vi "Crop Video Size Utility.vi"() -> ()   [LabVIEW 2017]
uses:
  LabVIEW/Controls/Frame Grabber Data.ctl
  <vilib>/userdefined/High Color/IMAQdx.ctl
  <vilib>/vision/Image Controls.llb/IMAQ Image.ctl
  <vilib>/vision/Avi.llb/IMAQ AVI2 Refnum.ctl
  LabVIEW/Controls/Rigid Body Info.ctl
  LabVIEW/Controls/Position.ctl
  LabVIEW/Controls/Orientation.ctl
  LabVIEW/Controls/Refnums.ctl
  LabVIEW/Controls/Recording Settings.ctl
  LabVIEW/Controls/Operator Settings.ctl
  LabVIEW/Controls/Operator.ctl
  LabVIEW/Controls/Dimensions.ctl
  LabVIEW/Controls/Room Dimensions.ctl
  <vilib>/vision/NI_Vision_Development_Module.lvlib
panel:
  in  "Codec":u16(ring)=3 items=["Cinepak Codec by Radius", "Intel IYUV codec", "Microsoft Video 1", "FF Video Codec 1 (FFV1) (NI Vision)", "Motion JPEG (NI Vision)", "Y800 Uncompressed Grey Scale (NI Vision)", "YUV 4:2:0 Planar (NI Vision)"]
  out "Saving":bool
  in  "Display While Saving?":bool
  in  "Crop":bool
  in  "Reset Crop":bool
  in  "Stop":bool
  out "Video path":path
  out "Crop ROI":i32[](array[numeric])
  in  "Frame Grabber Data":T1={"Camera Session"="", "Frame"=refnum, "AVI Refnum"=refnum, "Codecs"=[], "Frame number"=0, "Tracking File Refnum"=refnum, "Tick Count"=0, "Probe Object"=refnum, "Playback Probe Data"=[], "Rigid Body"={"Position"={"x (mm)"=0.0, "y (mm)"=0.0, "z (mm)"=0.0}, "Orientation"={"Pitch (rad)"=0.0, "Yaw (rad)"=0.0, "Roll (rad)"=0.0}, "Quaternion"={"qx"=0.0, "qy"=0.0, "qz"=0.0, "qw"=0.0}, "Tracked?"=FALSE}, "Total no frames playback"=0, "Video FPS"=0.0, "Camera connected?"=FALSE, "Scene"=refnum, "Cropped Frame"=refnum, "Tracker FPS"=0.0, "Crop ROI"=[], "Presentation Values"=[], "Elapsed time (ms)"=0, "Camera frames playback"=0, "Refnums"={"Live Refnum"=refnum, "Record Refnum"=refnum, "Recording Settings Refnum"=refnum, "Playback Refnum"=refnum, "Frame Slider Refnum"=refnum, "Pause Refnum"=refnum, "Home Refnum"=refnum, "Crop Refnum"=refnum, "Clear Crop Refnum"=refnum, "stop refnum"=refnum, "Playback Rate Refnum"=refnum, "Operator Settings Refnums"=refnum, "Presentation Refnum"=refnum, "Gestation Refnum"=refnum, "Connection Settings Refnum"=refnum, "Crop Time Frame Slider Refnum"=refnum}, "Dimensions"={"Probe Dimensions"={"Probe Width"=0.0, "Probe Depth"=1.0, "Probe Height"=0.0}, "Room Dimensions"={"Room Width"=0.0, "Room Depth"=0.0, "Room Height"=0.0}}, "Playback Data As Strings"=[], "Cropped Tracking File Refnum"=refnum, "Cropped AVI Refnum"=refnum, "Header"=[]}
  in  "Save":bool
  in  "Open":bool
  out "Frame":T3(plugin-control)
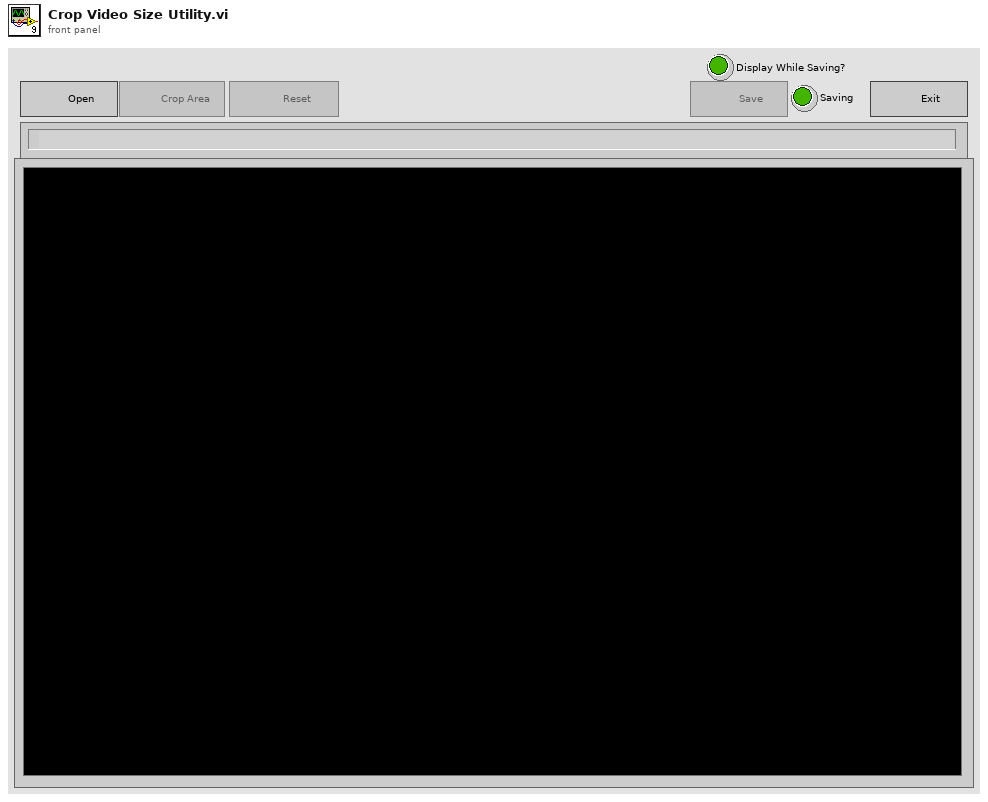
[diagram p1: front panel]
types:
  T1 = typedef "Frame Grabber Data.ctl" = cluster{"Camera Session":T2, "Frame":T3, "AVI Refnum":T4, "Codecs":string[], "Frame number":u32, "Tracking File Refnum":refnum<file>, "Tick Count":u32, "Probe Object":refnum<vi>, "Playback Probe Data":dbl[][], "Rigid Body":T5, "Total no frames playback":i32, "Video FPS":dbl, "Camera connected?":bool, "Scene":refnum<vi>, "Cropped Frame":T3, "Tracker FPS":dbl, "Crop ROI":i32[], "Presentation Values":string[], "Elapsed time (ms)":u32, "Camera frames playback":u32, "Refnums":T8, "Dimensions":T9, "Playback Data As Strings":string[][], "Cropped Tracking File Refnum":refnum<file>, "Cropped AVI Refnum":T4, "Header":string[]}
  T2 = typedef "IMAQdx.ctl" = refnum<k21>
  T3 = typedef "IMAQ Image.ctl" = refnum<image>
  T4 = typedef "IMAQ AVI2 Refnum.ctl" = refnum<k20>
  T5 = typedef "Rigid Body Info.ctl" = cluster{"Position":T6, "Orientation":T7, "Quaternion":cluster{"qx":sgl, "qy":sgl, "qz":sgl, "qw":sgl}, "Tracked?":bool}
  T6 = typedef "Position.ctl" = cluster{"x (mm)":sgl, "y (mm)":sgl, "z (mm)":sgl}
  T7 = typedef "Orientation.ctl" = cluster{"Pitch (rad)":sgl, "Yaw (rad)":sgl, "Roll (rad)":sgl}
  T8 = typedef "Refnums.ctl" = cluster{"Live Refnum":refnum<vi>, "Record Refnum":refnum<vi>, "Recording Settings Refnum":refnum<vi>, "Playback Refnum":refnum<vi>, "Frame Slider Refnum":refnum<vi>, "Pause Refnum":refnum<vi>, "Home Refnum":refnum<vi>, "Crop Refnum":refnum<vi>, "Clear Crop Refnum":refnum<vi>, "stop refnum":refnum<vi>, "Playback Rate Refnum":refnum<vi>, "Operator Settings Refnums":refnum<vi>, "Presentation Refnum":refnum<vi>, "Gestation Refnum":refnum<vi>, "Connection Settings Refnum":refnum<vi>, "Crop Time Frame Slider Refnum":refnum<vi>}
  T9 = typedef "Dimensions.ctl" = cluster{"Probe Dimensions":cluster{"Probe Width":sgl, "Probe Depth":sgl, "Probe Height":sgl}, "Room Dimensions":T10}
  T10 = typedef "Room Dimensions.ctl" = cluster{"Room Width":dbl, "Room Depth":dbl, "Room Height":dbl}
  T11 = enum8{"Enabled", "Disabled", "Disabled and Grayed Out"}
  T12 = typedef "Image Type" = u32
  T13 = enum16{"open", "replace", "create", "open or create", "replace or create", "replace or create with confirmation"}
  T14 = cluster{"Width":u32, "Height":u32, "Frames Per Second":u32, "Codec":string, "Has Data":bool}
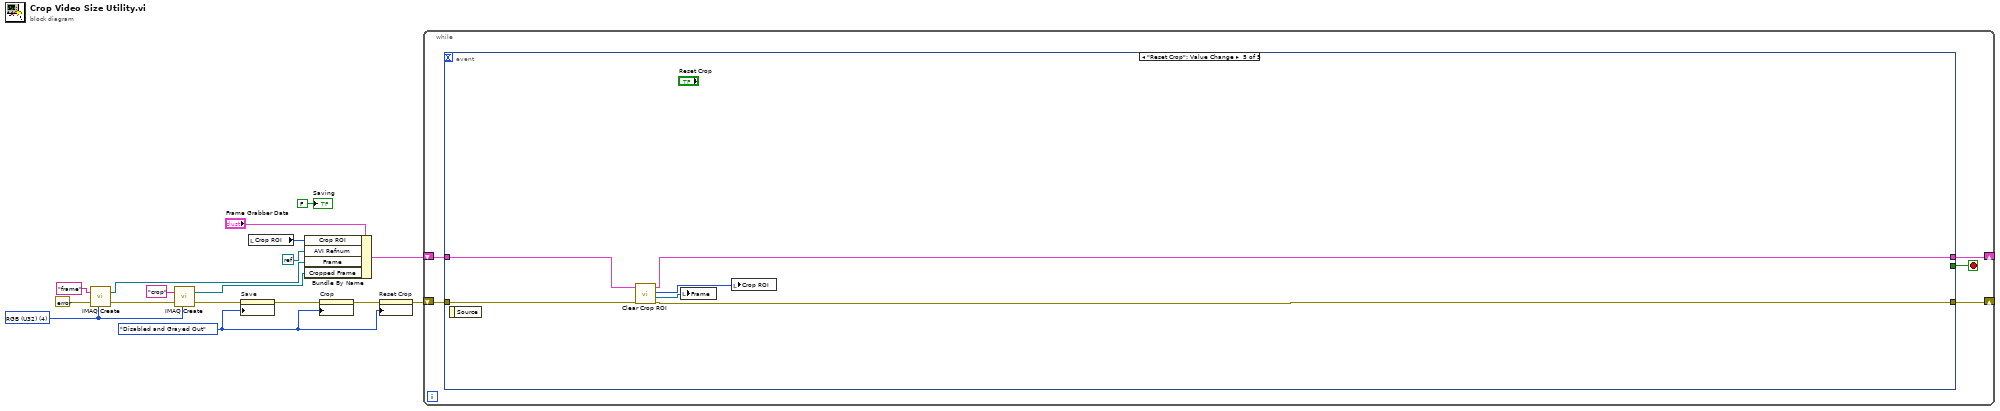
[diagram p0: block diagram]
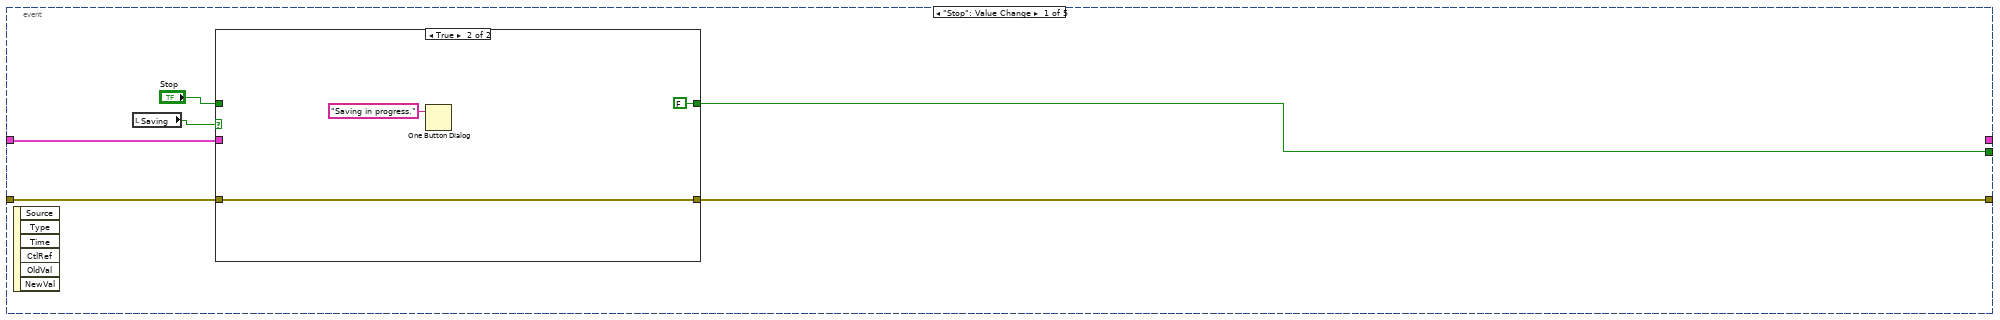
[diagram p2: hidden frame]
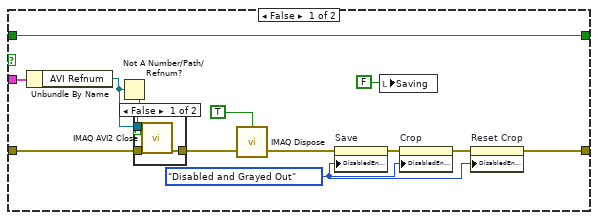
[diagram p3: hidden frame]
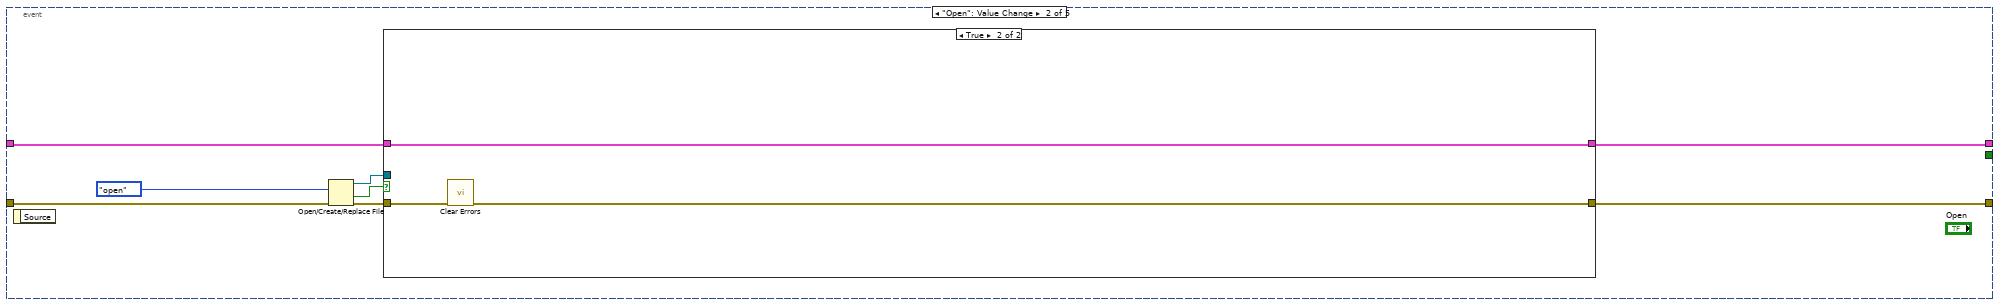
[diagram p5: hidden frame]
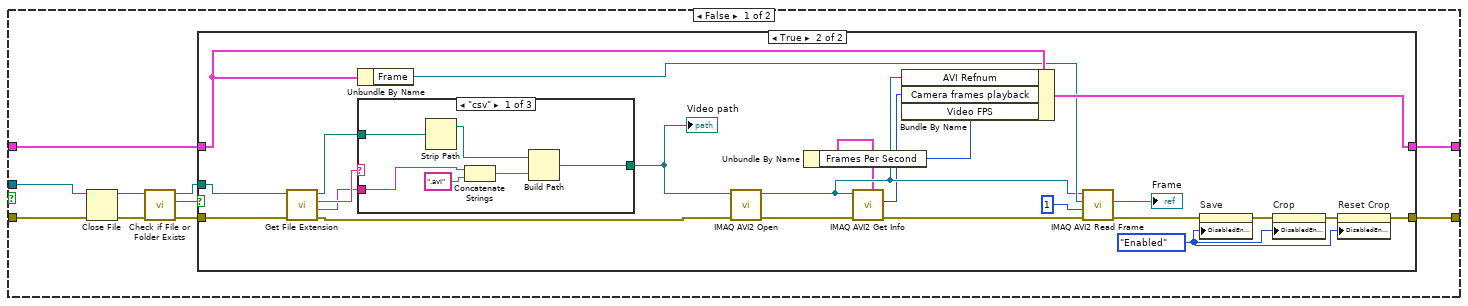
[diagram p6: hidden frame]
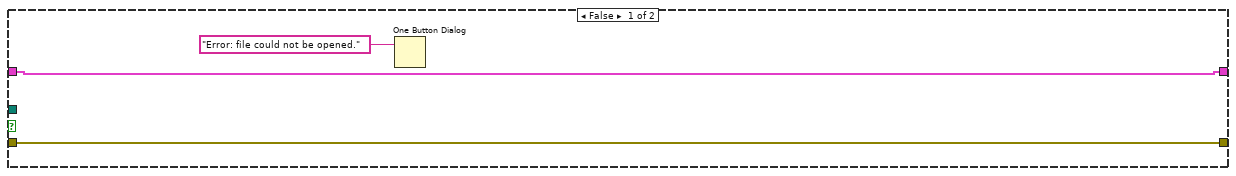
[diagram p7: hidden frame]
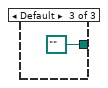
[diagram p9: hidden frame]
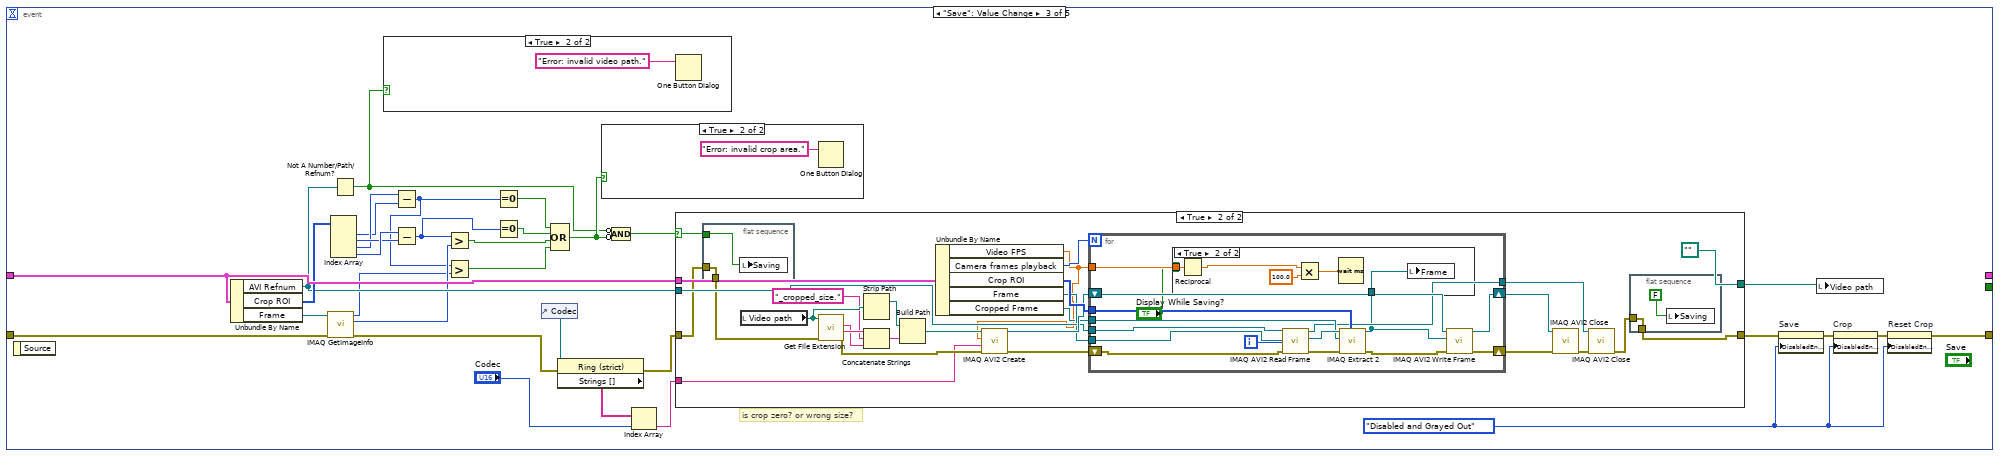
[diagram p10: hidden frame]
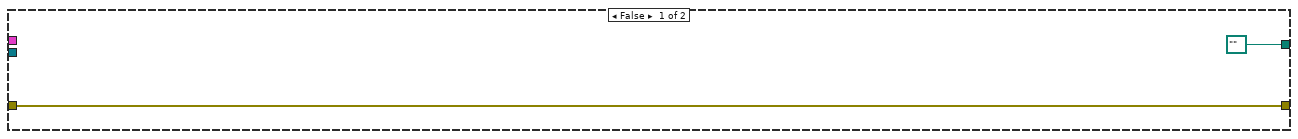
[diagram p13: hidden frame]
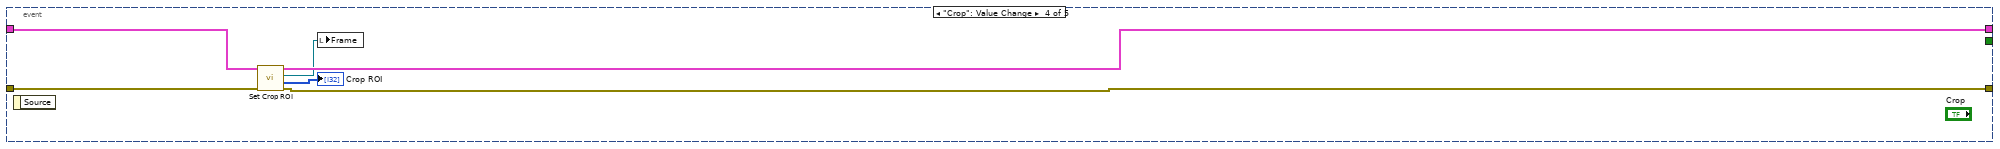
[diagram p15: hidden frame]
diagram:
  w2 = T11."Disabled and Grayed Out" ("Disabled")
  w9 = T12 4 items=["Grayscale (U8)", "Grayscale (I16)", "Grayscale (SGL)", "Complex (CSG)", "RGB (U32)", "HSL (U32)", "RGB (U64)", "Grayscale (U16)"] ("Image Type")
  n1 = call "IMAQ Create"("Image Name"="frame", "Image Type"=w9, "error in (no error)"=errorcluster {"status"=FALSE, "code"=0, "source"=""}) -> ("New Image"=w12:T3, "error out"=w10:errorcluster)  [unwired: 2 in]
  n2 = call "IMAQ Create"("Image Name"="crop", "Image Type"=w9, "error in (no error)"=w10) -> ("New Image"=w13:T3, "error out"=w6:errorcluster)  [unwired: 2 in]
  n3 = property on="Save" class="Bool"(error in=w6, "DisabledEnum"=w2) -> (error out=w5:errorcluster)  [unwired: 1 in, 1 out]
  n4 = local read "Crop ROI"() -> (w7:i32[])
  n5 = Bundle By Name(cluster="Frame Grabber Data", "Crop ROI"=w7, "AVI Refnum"=refnum<k0> refnum, "Frame"=w12, "Cropped Frame"=w13) -> (w16:T1)
  n6 = property on="Crop" class="Bool"(error in=w5, "DisabledEnum"=w2) -> (error out=w3:errorcluster)  [unwired: 1 in, 1 out]
  n7 = property on="Reset Crop" class="Bool"(error in=w3, "DisabledEnum"=w2) -> (error out=w4:errorcluster)  [unwired: 1 in, 1 out]
  n8 = while {
    shift-right: [w19] -> _
    shift-left: w16 -> [w20]
    shift-right: [w18] -> _
    shift-left: w4 -> [w21]
    stop <- w22 stop-if-true
    n9 = event shown="[4] \"Reset Crop\": Value Change" {
      selector: _ -> [_ _ _ _ _]
      dyn-events: _ -> [_ _ _ _ _]
      timeout: _ -> [_ _ _ _ _]
      tunnel: [w23 _ _ _ _] -> w22
      tunnel: w21 -> [w28 w56 w122 w197 w201]
      tunnel: w20 -> [w27 w51 w135 w198 w204]
      tunnel: [_ w50 _ w196 w199] -> w19
      tunnel: [w26 w49 w113 w193 w200] -> w18
      event "Stop": Value Change {
        n10 = event-data() -> ()  [unwired: 1 in, 6 out]
        n11 = local read "Saving"() -> (w24:bool)
        n12 = case shown="True" w24 {
          tunnel: w28 -> [w41 w47]
          tunnel: w27 -> [w40 _]
          tunnel: [w36 w47] -> w26
          tunnel: "Stop" -> [w29 _]
          tunnel: [w29 FALSE ("Stop")] -> w23
          frame False {
            w33 = T11."Disabled and Grayed Out" ("Disabled")
            n13 = Unbundle By Name(w40) -> ("AVI Refnum"=w31:T4)
            n14 = Not A Number/Path/Refnum?(number/path/refnum=w31) -> (NaN/Path/Refnum?=w30:bool)
            n15 = case shown="False" w30 {
              tunnel: w41 -> [w44 w45]
              tunnel: [w43 w45] -> w38
              tunnel: w31 -> [w42 _]
              frame False {
                n16 = call "IMAQ AVI2 Close"("error in (no error)"=w44, "AVI Refnum"=w42) -> ("error out"=w43:errorcluster)  [unwired: 9 in]
              }
              frame True {
              }
            }
            n17 = call "IMAQ Dispose"("All Images? (No)"=TRUE, "error in (no error)"=w38) -> ("error out"=w37:errorcluster)  [unwired: 4 in]
            n18 = property on="Save" class="Bool"(error in=w37, "DisabledEnum"=w33) -> (error out=w34:errorcluster)  [unwired: 1 in, 1 out]
            n19 = local write "Saving"(FALSE) -> ()
            n20 = property on="Crop" class="Bool"(error in=w34, "DisabledEnum"=w33) -> (error out=w35:errorcluster)  [unwired: 1 in, 1 out]
            n21 = property on="Reset Crop" class="Bool"(error in=w35, "DisabledEnum"=w33) -> (error out=w36:errorcluster)  [unwired: 1 in, 1 out]
          }
          frame True {
            n22 = One Button Dialog(message="Saving in progress.") -> ()  [unwired: 1 in, 1 out]
          }
        }
      }
      event "Open": Value Change {
        n23 = event-data() -> ()  [unwired: 1 in, 1 out]
        n24 = Open/Create/Replace File(error in=w56, operation (0:open)=T13."open") -> (refnum out=w52:refnum<file>, cancelled=w55:bool, error out=w53:errorcluster)  [unwired: 4 in]
        n25 = case shown="True" w55 {
          tunnel: w53 -> [w63 w102]
          tunnel: w52 -> [w64 _]
          tunnel: w51 -> [w60 w103]
          tunnel: [w59 w103] -> w50
          tunnel: [w57 w101] -> w49
          frame False {
            n26 = Close File(refnum=w64, error in=w63) -> (path=w61:path, error out=w62:errorcluster)
            n27 = call <vilib>:"Check if File or Folder Exists.vi"("error in (no error)"=w62, "path"=w61) -> ("error out"=w66:errorcluster, "file or folder exists?"=w58:bool, "dup path"=w65:path)  [unwired: 7 in]
            n28 = case shown="True" w58 {
              tunnel: w66 -> [w68 w78]
              tunnel: w65 -> [_ w74]
              tunnel: w60 -> [w69 w91]
              tunnel: [w69 w92] -> w59
              tunnel: [w68 w80] -> w57
              frame False {
                n29 = One Button Dialog(message="Error: file could not be opened.") -> ()  [unwired: 1 in, 1 out]
              }
              frame True {
                w79 = T11."Enabled" ("Disabled")
                n30 = call <vilib>:"Get File Extension.vi"("error in (no error)"=w78, "file"=w74) -> ("error out"=w77:errorcluster, "filename without extension"=w75:string, "lowercase file extension"=w76:string, "dup file"=w73:path)  [unwired: 5 in, 1 out]
                n31 = Unbundle By Name(w91) -> ("Frame"=w90:T3)
                n32 = case shown="\"csv\"" w76 {
                  tunnel: w75 -> [w98 _ _]
                  tunnel: [w93 w99 path "" ("dup file")] -> w72
                  tunnel: w73 -> [w94 w99 _]
                  frame "csv" {
                    n33 = Strip Path(path=w94) -> (stripped path=w96:path)  [unwired: 1 out]
                    n34 = Concatenate Strings(w98, ".avi" ("string")) -> (w95:string)
                    n35 = Build Path(base path=w96, name or relative path=w95) -> (appended path=w93:path)
                  }
                  frame "avi" {
                  }
                  frame Default {
                  }
                }
                "Video path" <- w72
                n36 = call "IMAQ AVI2 Open"("error in (no error)"=w77, "AVI File Path"=w72) -> ("error out"=w86:errorcluster, "AVI Refnum"=w87:T4)  [unwired: 8 in]
                n37 = call "IMAQ AVI2 Get Info"("error in (no error)"=w86, "AVI Refnum"=w87) -> ("error out"=w85:errorcluster, "Number of Frames"=w84:u32, "Frame Data"=w71:T14)  [unwired: 5 in, 2 out]
                n38 = Unbundle By Name(w71) -> ("Frames Per Second"=w70:u32)
                n39 = Bundle By Name(cluster=w91, "AVI Refnum"=w87, "Camera frames playback"=w84, "Video FPS"=w70) -> (w92:T1)
                n40 = call "IMAQ AVI2 Read Frame"("error in (no error)"=w85, "Frame Number"=u32 1, "Image"=w90, "AVI Refnum"=w87) -> ("error out"=w83:errorcluster, "Image Out"=→"Frame":T3)  [unwired: 5 in, 1 out]
                n41 = property on="Save" class="Bool"(error in=w83, "DisabledEnum"=w79) -> (error out=w82:errorcluster)  [unwired: 1 in, 1 out]
                n42 = property on="Crop" class="Bool"(error in=w82, "DisabledEnum"=w79) -> (error out=w81:errorcluster)  [unwired: 1 in, 1 out]
                n43 = property on="Reset Crop" class="Bool"(error in=w81, "DisabledEnum"=w79) -> (error out=w80:errorcluster)  [unwired: 1 in, 1 out]
              }
            }
          }
          frame True {
            n44 = call <vilib>:"Clear Errors.vi"("error in (no error)"=w102) -> ("error out"=w101:errorcluster)  [unwired: 5 in, 1 out]
          }
        }
      }
      event "Save": Value Change {
        w111 = T11."Disabled and Grayed Out" ("Disabled")
        # "is crop zero? or wrong size?"
        n45 = event-data() -> ()  [unwired: 1 in, 1 out]
        n46 = Unbundle By Name(w135) -> ("AVI Refnum"=w123:T4, "Crop ROI"=w128:i32[], "Frame"=w121:T3)
        n47 = call "IMAQ GetImageInfo"("error in (no error)"=w122, "Image"=w121) -> ("error out"=w110:errorcluster, "Y Resolution"=w120:i32, "X Resolution"=w118:i32)  [unwired: 2 in, 5 out]
        n48 = Index Array(array=w128) -> (element #1=w129:i32, element #2=w131:i32, element #3=w130:i32, element #4=w132:i32)  [unwired: 4 in]
        n49 = Not A Number/Path/Refnum?(number/path/refnum=w123) -> (NaN/Path/Refnum?=w124:bool)
        n50 = case shown="True" w124 {
          frame False {
          }
          frame True {
            n51 = One Button Dialog(message="Error: invalid video path.") -> ()  [unwired: 1 in, 1 out]
          }
        }
        n52 = Subtract(x=w130, y=w129) -> (x-y=w117:i32)
        n53 = Subtract(x=w132, y=w131) -> (x-y=w115:i32)
        n54 = Greater?(x=w115, y=w120) -> (0:w119:bool)
        n55 = Greater?(x=w117, y=w118) -> (0:w116:bool)
        n56 = Equal To 0?(x=w117) -> (x = 0?=w133:bool)
        n57 = Equal To 0?(x=w115) -> (x = 0?=w134:bool)
        n58 = control-ref of="Codec"() -> (w108:refnum<vi>)
        n59 = Compound Arithmetic op=OR(w133, w134, w119, w116) -> (w125:bool)
        n60 = property class="Ring (strict)"(reference=w108, error in=w110) -> (error out=w109:errorcluster, "Strings []"=w106:string[])  [unwired: 1 out]
        n61 = case shown="True" w125 {
          frame False {
          }
          frame True {
            n62 = One Button Dialog(message="Error: invalid crop area.") -> ()  [unwired: 1 in, 1 out]
          }
        }
        n63 = Compound Arithmetic op=AND(invert w124, invert w125) -> (w126:bool)
        n64 = Index Array(array=w106, index="Codec") -> (element=w105:string)
        n65 = case shown="True" w126 {
          selector: w126 -> [_ w147]
          tunnel: w135 -> [_ w167]
          tunnel: w123 -> [_ w154]
          tunnel: [w139 w143] -> w127
          tunnel: w109 -> [w139 w146]
          tunnel: w105 -> [_ w142]
          tunnel: [path "" ("Video path") path "" ("Video path")] -> w104
          frame False {
          }
          frame True {
            n66 = flat-sequence {
              tunnel: w147 -> [w171]
              tunnel: w146 -> [w170]
              tunnel: [w170] -> w145
              frame #0 {
                n67 = local write "Saving"(w171) -> ()
              }
            }
            n68 = local read "Video path"() -> (w162:path)
            n69 = call <vilib>:"Get File Extension.vi"("error in (no error)"=w145, "file"=w162) -> ("error out"=w163:errorcluster, "filename without extension"=w160:string, "lowercase file extension"=w158:string)  [unwired: 5 in, 2 out]
            n70 = Strip Path(path=w162) -> (stripped path=w161:path)  [unwired: 1 out]
            n71 = Concatenate Strings(w160, "_cropped_size." ("string"), w158) -> (w157:string)
            n72 = Build Path(base path=w161, name or relative path=w157) -> (appended path=w156:path)
            n73 = Unbundle By Name(w167) -> ("Video FPS"=w141:dbl, "Camera frames playback"=w166:u32, "Crop ROI"=w165:i32[], "Frame"=w153:T3, "Cropped Frame"=w152:T3)
            n74 = call "IMAQ AVI2 Create"("error in (no error)"=w163, "Codec"=w142, "Frames Per Second"=w141, "AVI Path"=w156) -> ("error out"=w155:errorcluster, "AVI Refnum"=w164:T4)  [unwired: 6 in]
            n75 = for {
              N: w166 -> [_]
              shift-right: [w182] -> w151
              shift-left: w155 -> [w186]
              tunnel: w165 -> [w185]
              tunnel: w154 -> [w181]
              tunnel: w153 -> [w180]
              tunnel: w152 -> [w178]
              shift-right: [w177] -> w150
              shift-left: w164 -> [w184]
              tunnel: [w176] -> w148
              tunnel: w141 -> [w173]
              i -> [w187]
              n76 = call "IMAQ AVI2 Read Frame"("error in (no error)"=w186, "Frame Number"=w187, "Image"=w180, "AVI Refnum"=w181) -> ("error out"=w174:errorcluster, "Image Out"=w179:T3, "AVI Refnum (duplicate)"=w176:T4)  [unwired: 5 in]
              n77 = call "IMAQ Extract 2"("Optional Rectangle"=w185, "error in (no error)"=w174, "Image Dst"=w178, "Image Src"=w179) -> ("error out"=w183:errorcluster, "Image Dst Out"=w175:T3)  [unwired: 6 in]
              n78 = case shown="True" "Display While Saving?" {
                tunnel: w175 -> [_ w192]
                tunnel: w173 -> [_ w191]
                frame False {
                }
                frame True {
                  n79 = Reciprocal(x=w191) -> (1/x=w190:dbl)
                  n80 = Multiply(x=w190, y=100.0) -> (x*y=w188:dbl)
                  n81 = Wait (ms)(milliseconds to wait=w188) -> ()  [unwired: 1 out]
                  n82 = local write "Frame"(w192) -> ()
                }
              }
              n83 = call "IMAQ AVI2 Write Frame"("error in (no error)"=w183, "Image"=w175, "AVI Refnum"=w184) -> ("error out"=w182:errorcluster, "AVI Refnum (duplicate)"=w177:T4)  [unwired: 6 in, 1 out]
            }
            n84 = call "IMAQ AVI2 Close"("error in (no error)"=w151, "AVI Refnum"=w150) -> ("error out"=w149:errorcluster)  [unwired: 9 in]
            n85 = call "IMAQ AVI2 Close"("error in (no error)"=w149, "AVI Refnum"=w148) -> ("error out"=w144:errorcluster)  [unwired: 9 in]
            n86 = flat-sequence {
              tunnel: w144 -> [w169]
              tunnel: [w169] -> w143
              frame #0 {
                n87 = local write "Saving"(FALSE) -> ()
              }
            }
          }
        }
        n88 = property on="Save" class="Bool"(error in=w127, "DisabledEnum"=w111) -> (error out=w112:errorcluster)  [unwired: 1 in, 1 out]
        n89 = local write "Video path"(w104) -> ()
        n90 = property on="Crop" class="Bool"(error in=w112, "DisabledEnum"=w111) -> (error out=w114:errorcluster)  [unwired: 1 in, 1 out]
        n91 = property on="Reset Crop" class="Bool"(error in=w114, "DisabledEnum"=w111) -> (error out=w113:errorcluster)  [unwired: 1 in, 1 out]
      }
      event "Crop": Value Change {
        n92 = event-data() -> ()  [unwired: 1 in, 1 out]
        n93 = call "Set Crop ROI.vi"("error in (no error)"=w197, "Frame Grabber Data in"=w198) -> ("error out"=w193:errorcluster, "Crop ROI"=→"Crop ROI":i32[], "Image Out"=w195:T3, "Frame Grabber Data out"=w196:T1)  [unwired: 5 in, 1 out]
        n94 = local write "Frame"(w195) -> ()
      }
      event "Reset Crop": Value Change {
        n95 = event-data() -> ()  [unwired: 1 in, 1 out]
        n96 = call "Clear Crop ROI.vi"("error in (no error)"=w201, "Frame Grabber Data in"=w204) -> ("error out"=w200:errorcluster, "Image Out"=w203:T3, "Crop ROI"=w202:i32[], "Frame Grabber Data out"=w199:T1)  [unwired: 6 in]
        n97 = local write "Frame"(w203) -> ()
        n98 = local write "Crop ROI"(w202) -> ()
      }
    }
  }
  "Saving" <- FALSE ("Saving")
